vi "HMI_main.vi"() -> ()   [LabVIEW 2018]
uses:
  <vilib>/RAFA Solutions/Harmony UI Controls Kit/String & Path/String Indicator.ctl
  <vilib>/RAFA Solutions/Harmony UI Controls Kit/Boolean/Slide Switch Round.ctl
  Controls/Cluster_HMI_VIFP - 2.ctl
  <vilib>/RAFA Solutions/Harmony UI Controls Kit/Numeric/Horizontal Progress Bar.ctl
  <vilib>/RAFA Solutions/Harmony UI Controls Kit/Numeric/Numeric Indicator.ctl
  <vilib>/RAFA Solutions/Harmony UI Controls Kit/Boolean/Blank Button - Blue.ctl
  <vilib>/RAFA Solutions/Harmony UI Controls Kit/Boolean/Blank Button - Red.ctl
  <vilib>/RAFA Solutions/Harmony UI Controls Kit/Boolean/Blank Button - Grey.ctl
  Controls/Hora y Fecha control.ctl
  Global/MSG.vi
  Global/datos usuario.vi
  <vilib>/addons/database/Connection.llb/DB Tools Open Connec (Path).vi
  Global/estadoGeneradores.vi
  Global/Alarmas_indicadores-LED.vi
  Global/globalEventos.vi
  Global/Demo.vi
  Global/globalGenerador1_HMI.vi
  Global/globalGenerador2_HMI.vi
  Global/globalGenerador3_HMI.vi
  Global/globalGenerador4_HMI.vi
  Global/globalGenerador5_HMI.vi
  Global/globalGenerador6_HMI.vi
  <vilib>/addons/database/NI_Database_API.lvlib
  <vilib>/RAFA Solutions/Harmony UI Controls Kit/Flat UI Design.lvlib
panel:
  out "build":string
  out "fecha y hora":T1
  in  "type specifier VI Refnum (for type only) 3":refnum<vi>
  in  "web_equipo":T2
  in  "type specifier VI Refnum (for type only) 2":refnum<vi>
  out "G6_TRANS":bool caption="Transiente"
  out "G6_SWELL":bool caption="Swell"
  out "G6_SAG":bool caption="Sag"
  out "G5_TRANS":bool caption="Transiente"
  out "G5_SWELL":bool caption="Swell"
  out "G5_SAG":bool caption="Sag"
  out "G4_TRANS":bool caption="Transiente"
  out "G4_SWELL":bool caption="Swell"
  out "G4_SAG":bool caption="Sag"
  out "G3_TRANS":bool caption="Transiente"
  out "G3_SWELL":bool caption="Swell"
  out "G3_SAG":bool caption="Sag"
  out "G2_TRANS":bool caption="Transiente"
  out "G2_SWELL":bool caption="Swell"
  out "G2_SAG":bool caption="Sag"
  out "G1_TRANS":bool caption="Transiente"
  out "G1_SWELL":bool caption="Swell"
  out "G1_SAG":bool caption="Sag"
  in  "type specifier VI Refnum (for type only)":refnum<vi>
  in  "type specifier VI Refnum (for type only)":refnum<vi>
  in  "type specifier VI Refnum (for type only)":refnum<vi>
  in  "configuraciones":T2
  in  "historicos":T2
  in  "eventos":T2
  in  "alarmas":T2
  in  "salir":T3
  in  "type specifier VI Refnum (for type only)":refnum<vi>
  in  "Boolean 6":T4 caption="EMCE_W02"
  out "Estado 6":T5
  in  "Boolean 5":T4 caption="EMCE_W01"
  out "Estado 5":T5
  in  "Boolean 4":T4 caption="EMCE_G04"
  out "Estado 4":T5
  in  "Boolean 3":T4 caption="EMCE_G03"
  out "Estado 3":T5
  in  "Boolean 2":T4 caption="EMCE_G02"
  out "Estado 2":T5
  in  "Boolean 1":T4 caption="EMCE_G01"
  out "Estado 1":T5
  in  "EMCE W02":T6
  in  "EMCE W01":T6
  in  "EMCE G04":T6
  in  "EMCE G03":T6
  in  "EMCE G02":T6
  in  "EMCE G01":T6
  out "Generador6":T7 {"I1" scale=0.0..1200.0; "L1" scale=0.0..600.0; "Factor de Potencia" format="%#.1f"; "Potencia Total [kW]" format="%#.1f"; "Frecuencia [Hz]" format="%#.1f"; "I3" scale=0.0..1200.0; "I2" scale=0.0..1200.0; "L3" scale=0.0..600.0; "L2" scale=0.0..600.0}
  out "Generador5":T7 {"I1" scale=0.0..1200.0; "L1" scale=0.0..600.0; "Factor de Potencia" format="%#.1f"; "Potencia Total [kW]" format="%#.1f"; "Frecuencia [Hz]" format="%#.1f"; "I3" scale=0.0..1200.0; "I2" scale=0.0..1200.0; "L3" scale=0.0..600.0; "L2" scale=0.0..600.0}
  out "Generador4":T7 {"I1" scale=0.0..1200.0; "L1" scale=0.0..600.0; "Factor de Potencia" format="%#.1f"; "Potencia Total [kW]" format="%#.1f"; "Frecuencia [Hz]" format="%#.1f"; "I3" scale=0.0..1200.0; "I2" scale=0.0..1200.0; "L3" scale=0.0..600.0; "L2" scale=0.0..600.0}
  out "Generador3":T7 {"I1" scale=0.0..1200.0; "L1" scale=0.0..600.0; "Factor de Potencia" format="%#.1f"; "Potencia Total [kW]" format="%#.1f"; "Frecuencia [Hz]" format="%#.1f"; "I3" scale=0.0..1200.0; "I2" scale=0.0..1200.0; "L3" scale=0.0..600.0; "L2" scale=0.0..600.0}
  out "Generador2":T7 {"I1" scale=0.0..1200.0; "L1" scale=0.0..600.0; "Factor de Potencia" format="%#.1f"; "Potencia Total [kW]" format="%#.1f"; "Frecuencia [Hz]" format="%#.1f"; "I3" scale=0.0..1200.0; "I2" scale=0.0..1200.0; "L3" scale=0.0..600.0; "L2" scale=0.0..600.0}
  out "Generador1":T7 {"I1" scale=0.0..1200.0; "L1" scale=0.0..600.0; "Factor de Potencia" format="%#.1f"; "Potencia Total [kW]" format="%#.1f"; "Frecuencia [Hz]" format="%#.1f"; "I3" scale=0.0..1200.0; "I2" scale=0.0..1200.0; "L3" scale=0.0..600.0; "L2" scale=0.0..600.0}
  out "Eventos":T5
  # "SMCE"
  # "Sistema de Monitoreo de Calidad de Energía"
  # "POPA"
  # "PROA"
  # "K2"
  # "K1"
  # "RK2"
  # "RK1"
  # "VOLTAJES [Vrms]"
  # "CORRIENTES [Arms]"
  # "VOLTAJES [Vrms]"
  # "CORRIENTES [Arms]"
  # "VOLTAJES [Vrms]"
  # "CORRIENTES [Arms]"
  # "VOLTAJES [Vrms]"
  # "CORRIENTES [Arms]"
  # "VOLTAJES [Vrms]"
  # "CORRIENTES [Arms]"
  # "VOLTAJES [Vrms]"
  # "CORRIENTES [Arms]"
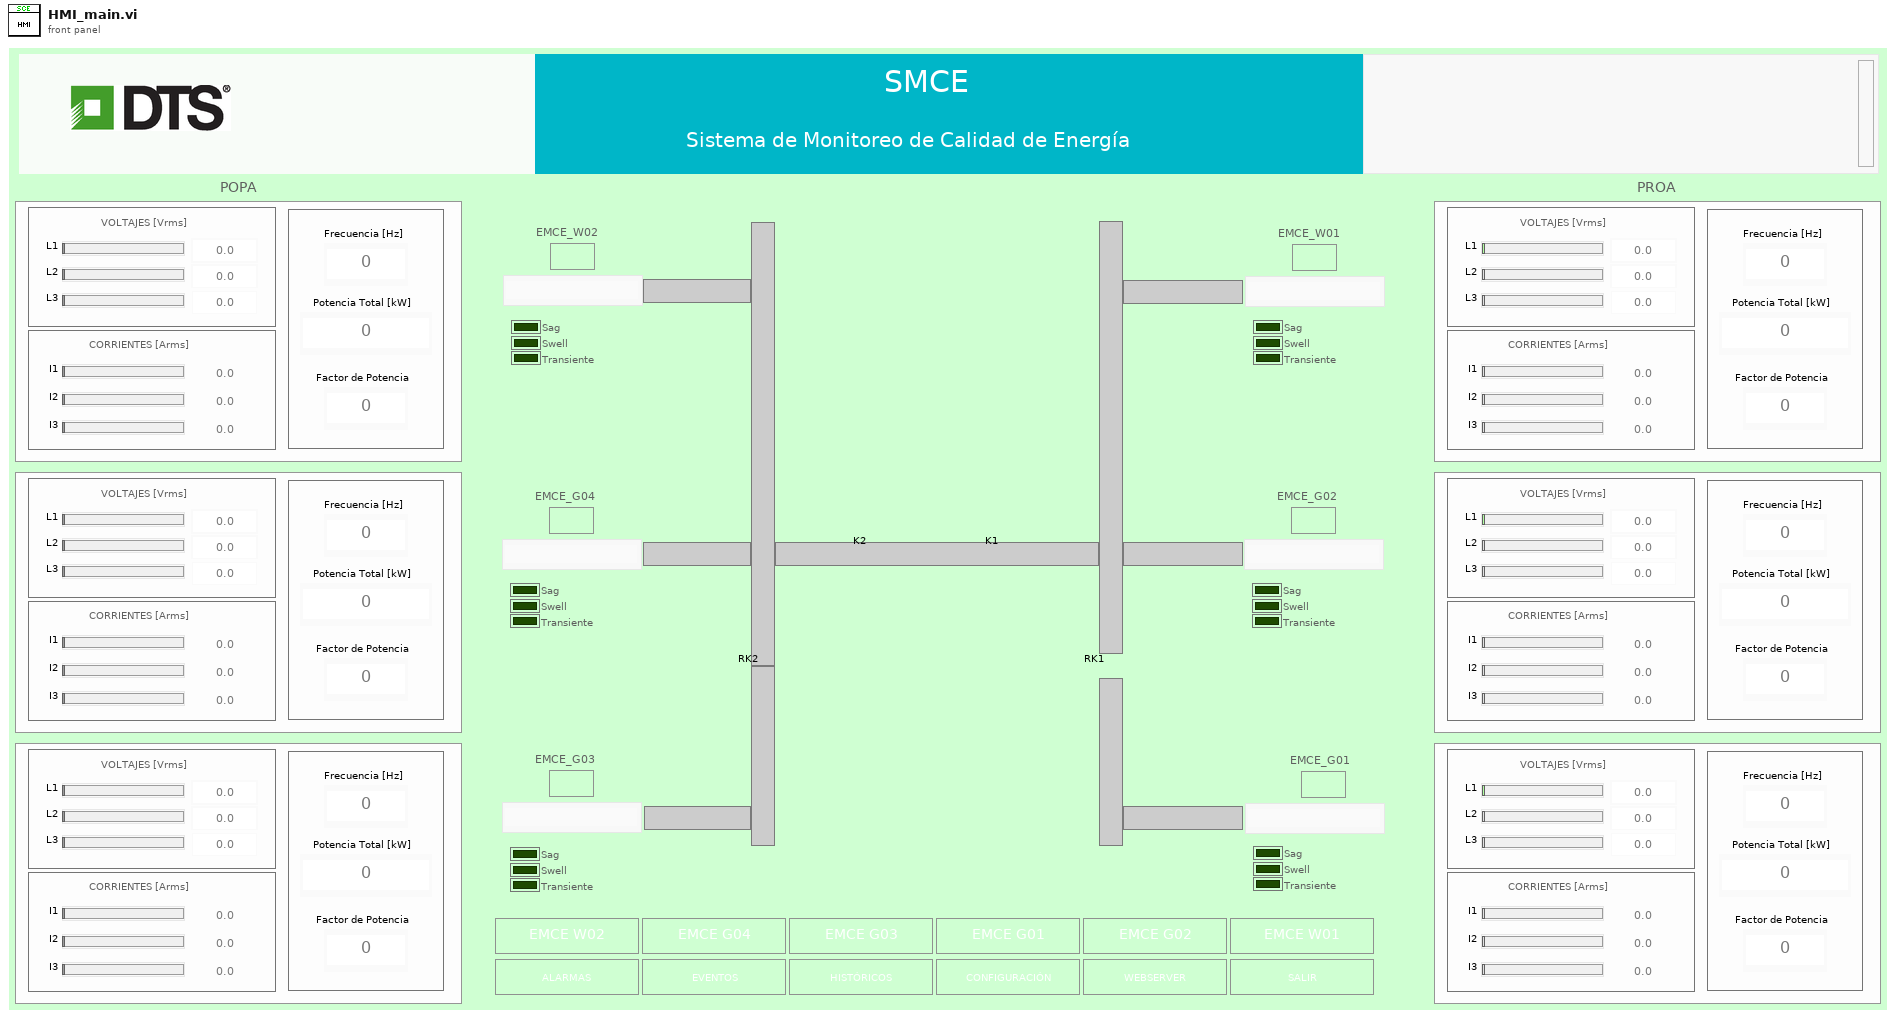
[diagram p1: front panel]
types:
  T1 = typedef "Hora y Fecha control.ctl" = cluster{"fecha":string, "dia semana":string, "fecha 2":string}
  T2 = typedef "Flat UI Design.lvlib/Blank Button - Grey.ctl" = bool
  T3 = typedef "Flat UI Design.lvlib/Blank Button - Red.ctl" = bool
  T4 = typedef "Flat UI Design.lvlib/Slide Switch Round.ctl" = bool
  T5 = typedef "Flat UI Design.lvlib/String Indicator.ctl" = string
  T6 = typedef "Flat UI Design.lvlib/Blank Button - Blue.ctl" = bool
  T7 = typedef "Cluster_HMI_VIFP - 2.ctl" = cluster{"L2":T8, "L3":T8, "I2":T8, "I3":T8, "Frecuencia [Hz]":T9, "Potencia Total [kW]":T9, "Factor de Potencia":T9, "L1":T8, "I1":T8}
  T8 = typedef "Flat UI Design.lvlib/Horizontal Progress Bar.ctl" = sgl
  T9 = typedef "Flat UI Design.lvlib/Numeric Indicator.ctl" = sgl
  T10 = enum8{"Enabled", "Disabled", "Disabled and Grayed Out"}
  T11 = typedef "NI_Database_API.lvlib/Conn ObjectReference.ctl" = refnum<k1>
  T12 = typedef "Equipos_Medicion_cluster.ctl" = cluster{"ID_EQUIPO":i32, "IP_EQUIPO":string, "NOMBRE_EQUIPO":string, "ESTADO_EQUIPO":string, "DESCRIPCION":string, "ID_MEDICION":i32, "ESTADO_MEDICION":string, "TIEMPO_MEDICION":string}
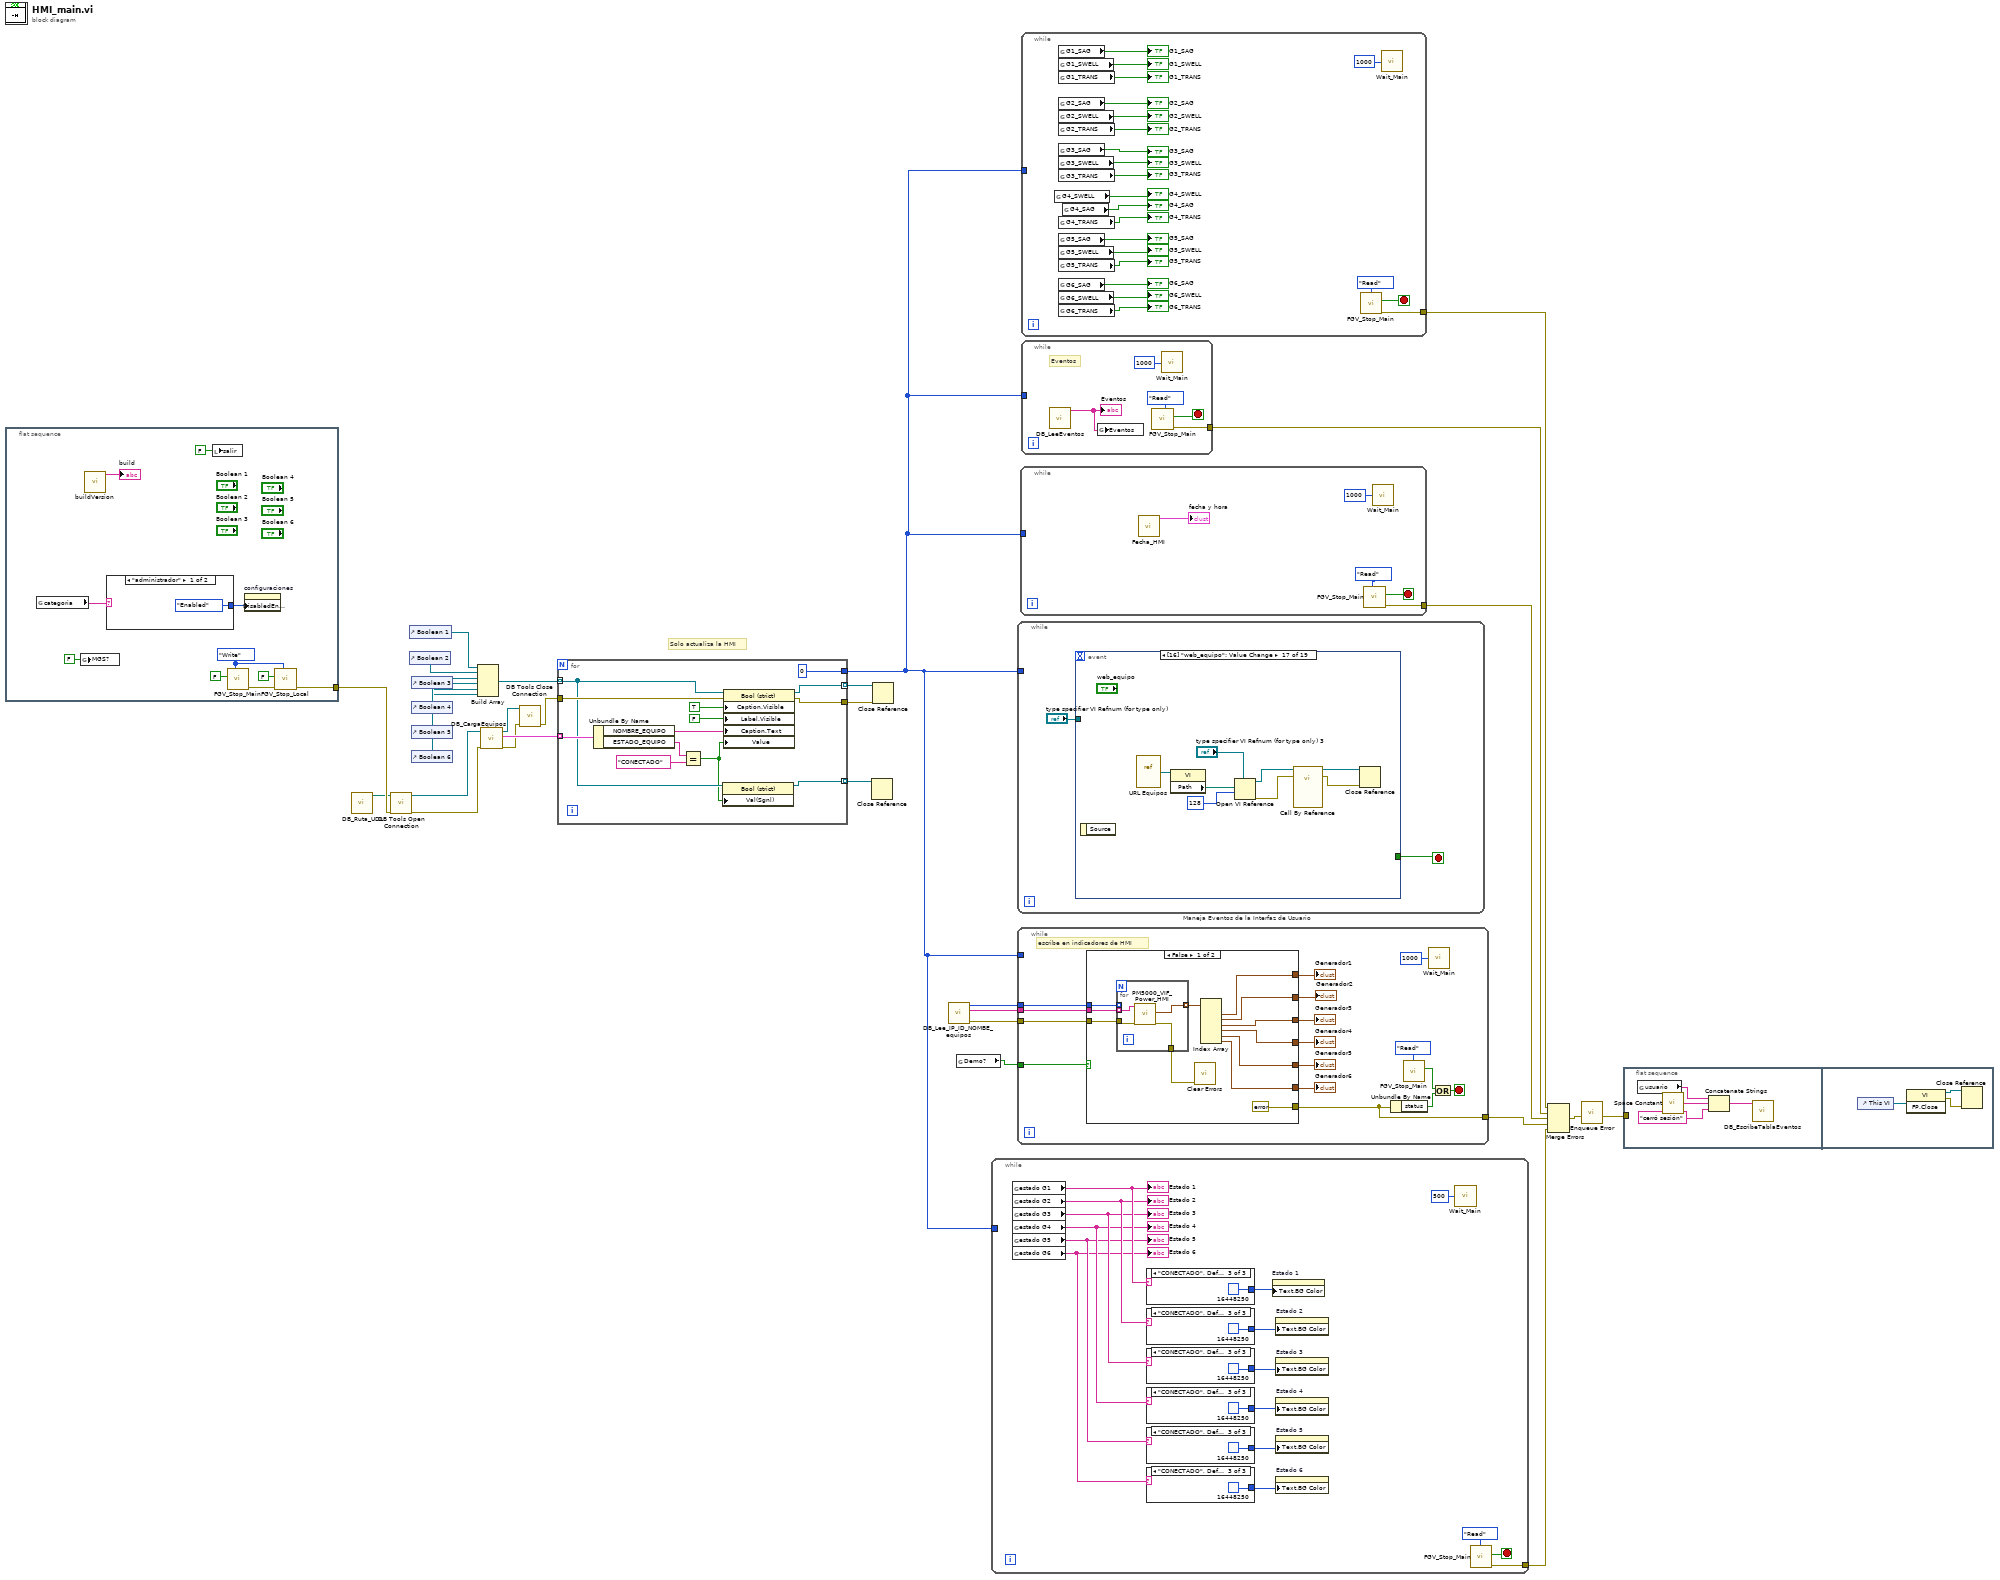
[diagram p0: block diagram]
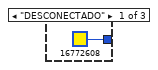
[diagram p2: hidden frame]
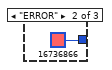
[diagram p3: hidden frame]
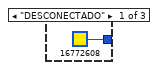
[diagram p4: hidden frame]
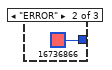
[diagram p5: hidden frame]
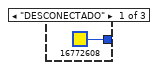
[diagram p6: hidden frame]
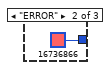
[diagram p7: hidden frame]
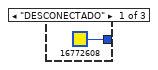
[diagram p8: hidden frame]
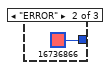
[diagram p9: hidden frame]
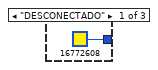
[diagram p10: hidden frame]
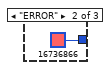
[diagram p11: hidden frame]
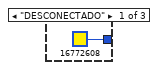
[diagram p12: hidden frame]
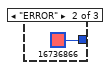
[diagram p13: hidden frame]
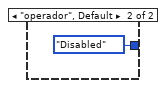
[diagram p14: hidden frame]
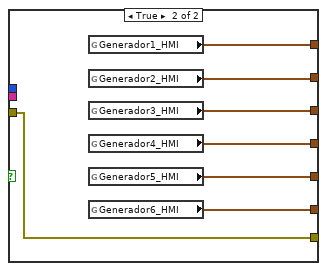
[diagram p15: hidden frame]
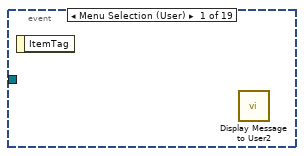
[diagram p16: hidden frame]
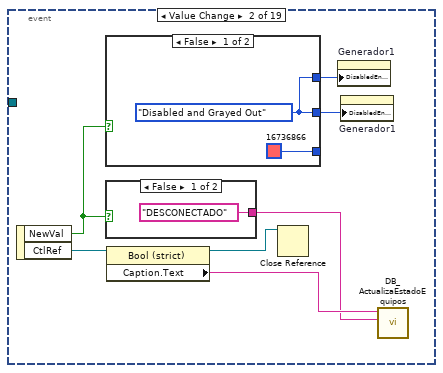
[diagram p17: hidden frame]
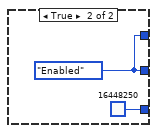
[diagram p18: hidden frame]
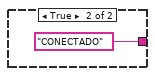
[diagram p19: hidden frame]
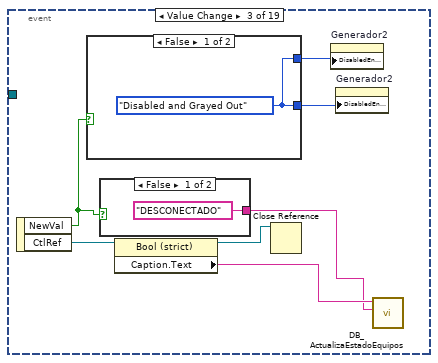
[diagram p20: hidden frame]
diagram:
  # "Solo actualiza la HMI"
  n1 = flat-sequence {
    tunnel: [w35] -> w19
    frame #0 {
      w38 = enum16{"Read", "Write"}."Write" ("Action")
      n2 = global read "datos usuario.vi" "categoria"() -> (w33:string)
      n3 = global write "MSG.vi" "MGS?"(FALSE ("MGS?")) -> ()
      n4 = call "buildVersion.vi"() -> ("build"=→"build":string)  [unwired: 11 in]
      n5 = case shown="\"administrador\"" w33 {
        tunnel: [T10."Enabled" ("Disabled") T10."Disabled" ("Disabled")] -> w34
        frame "administrador" {
        }
        frame "operador", Default {
        }
      }
      n6 = local write "salir"(T3 FALSE ("salir")) -> ()
      n7 = call "FGV_Stop_Main.vi"("Action"=w38, "Var In"=FALSE) -> ("Error Out"=w39:errorcluster)  [unwired: 8 in, 1 out]
      n8 = property on="configuraciones" class="Bool"("DisabledEnum"=w34) -> ()  [unwired: 2 in, 2 out]
      n9 = call "FGV_Stop_Local.vi"("Action"=w38, "Error In (no error)"=w39, "Var In"=FALSE) -> ("Error Out"=w35:errorcluster)  [unwired: 7 in, 1 out]
    }
  }
  n10 = call "DB_Ruta_UDL.vi"() -> ("UDL ruta"=w18:path)  [unwired: 11 in]
  n11 = call-poly <vilib>:"DB Tools Open Connection.vi"("error in (no error)"=w19, "connection information"=w18) -> ("error out"=w21:errorcluster, "connection reference"=w22:T11)  [unwired: 6 in]
  n12 = control-ref of="Boolean 2"() -> (w30:refnum<vi>)
  n13 = control-ref of="Boolean 1"() -> (w24:refnum<vi>)
  n14 = control-ref of="Boolean 3"() -> (w29:refnum<vi>)
  n15 = control-ref of="Boolean 4"() -> (w28:refnum<vi>)
  n16 = control-ref of="Boolean 5"() -> (w27:refnum<vi>)
  n17 = control-ref of="Boolean 6"() -> (w26:refnum<vi>)
  n18 = Build Array(w24, w30, w29, w28, w27, w26) -> (w25:refnum<vi>[])
  n19 = call "DB_CargaEquipos.vi"("error in (no error)"=w21, "db in"=w22) -> ("error out"=w12:errorcluster, "Equipos_out"=w23:T12[], "db out"=w20:T11)  [unwired: 2 in, 5 out]
  n20 = call <vilib>:"DB Tools Close Connection.vi"("error in (no error)"=w12, "connection reference"=w20) -> ("error out"=w11:errorcluster)  [unwired: 5 in]
  n21 = for {
    tunnel: w23 -> [w52] mode=indexing
    tunnel: w25 -> [w45] mode=indexing
    tunnel: [0] -> w2
    tunnel: [w50] -> w17
    tunnel: [w49] -> w16 mode=indexing
    tunnel: w11 -> [w48]
    tunnel: [w43] -> w4 mode=indexing
    n22 = Unbundle By Name(w52) -> ("NOMBRE_EQUIPO"=w47:string, "ESTADO_EQUIPO"=w46:string)
    n23 = Equal?(x=w46, y="CONECTADO") -> (x = y?=w44:bool)
    n24 = property class="Bool (strict)"(reference=w45, "Val(Sgnl)"=w44) -> (reference out=w43:refnum<vi>)  [unwired: 1 in, 1 out]
    n25 = property class="Bool (strict)"(reference=w45, error in=w48, "Caption.Visible"=TRUE ("Label.Visible"), "Label.Visible"=FALSE ("Caption.Visible"), "Caption.Text"=w47, "Value"=w44) -> (reference out=w49:refnum<vi>, error out=w50:errorcluster)
  }
  n26 = Close Reference(reference=w4) -> ()  [unwired: 1 in, 1 out]
  n27 = Close Reference(reference=w16, error in (no error)=w17) -> ()  [unwired: 1 out]
  n28 = call "DB_Lee_IP_ID_NOMBE_equipos.vi"() -> ("error out"=w15:errorcluster, "IP_EQUIPO"=w14:string[], "ID_EQUIPO"=w13:i32[])  [unwired: 8 in, 1 out]
  n29 = global read "Demo.vi" "Demo?"() -> (w1:bool)
  n30 = while {
    tunnel: [w56] -> w3
    tunnel: w2 -> [_]
    stop <- w70 stop-if-true
    n31 = global read "estadoGeneradores.vi" "estado G1"() -> (w68:string)
    "Estado 1" <- w68
    n32 = global read "estadoGeneradores.vi" "estado G2"() -> (w66:string)
    "Estado 2" <- w66
    n33 = global read "estadoGeneradores.vi" "estado G3"() -> (w65:string)
    "Estado 3" <- w65
    n34 = global read "estadoGeneradores.vi" "estado G4"() -> (w64:string)
    "Estado 4" <- w64
    n35 = global read "estadoGeneradores.vi" "estado G5"() -> (w63:string)
    "Estado 5" <- w63
    n36 = global read "estadoGeneradores.vi" "estado G6"() -> (w62:string)
    "Estado 6" <- w62
    n37 = case shown="\"CONECTADO\", Default" w68 {
      tunnel: [u32 16772608 u32 16736866 u32 16448250] -> w67
      frame "DESCONECTADO" {
      }
      frame "ERROR" {
      }
      frame "CONECTADO", Default {
      }
    }
    n38 = case shown="\"CONECTADO\", Default" w66 {
      tunnel: [u32 16772608 u32 16736866 u32 16448250] -> w61
      frame "DESCONECTADO" {
      }
      frame "ERROR" {
      }
      frame "CONECTADO", Default {
      }
    }
    n39 = case shown="\"CONECTADO\", Default" w65 {
      tunnel: [u32 16772608 u32 16736866 u32 16448250] -> w60
      frame "DESCONECTADO" {
      }
      frame "ERROR" {
      }
      frame "CONECTADO", Default {
      }
    }
    n40 = case shown="\"CONECTADO\", Default" w64 {
      tunnel: [u32 16772608 u32 16736866 u32 16448250] -> w59
      frame "DESCONECTADO" {
      }
      frame "ERROR" {
      }
      frame "CONECTADO", Default {
      }
    }
    n41 = case shown="\"CONECTADO\", Default" w63 {
      tunnel: [u32 16772608 u32 16736866 u32 16448250] -> w58
      frame "DESCONECTADO" {
      }
      frame "ERROR" {
      }
      frame "CONECTADO", Default {
      }
    }
    n42 = case shown="\"CONECTADO\", Default" w62 {
      tunnel: [u32 16772608 u32 16736866 u32 16448250] -> w57
      frame "DESCONECTADO" {
      }
      frame "ERROR" {
      }
      frame "CONECTADO", Default {
      }
    }
    n43 = property on="Estado 1" class="Str (strict)"("Text.BG Color"=w67) -> ()  [unwired: 2 in, 2 out]
    n44 = property on="Estado 2" class="Str (strict)"("Text.BG Color"=w61) -> ()  [unwired: 2 in, 2 out]
    n45 = property on="Estado 3" class="Str (strict)"("Text.BG Color"=w60) -> ()  [unwired: 2 in, 2 out]
    n46 = property on="Estado 4" class="Str (strict)"("Text.BG Color"=w59) -> ()  [unwired: 2 in, 2 out]
    n47 = property on="Estado 5" class="Str (strict)"("Text.BG Color"=w58) -> ()  [unwired: 2 in, 2 out]
    n48 = property on="Estado 6" class="Str (strict)"("Text.BG Color"=w57) -> ()  [unwired: 2 in, 2 out]
    n49 = call "Wait_Main.vi"("Wait time (msec)"=u32 500 ("milliseconds to wait")) -> ()  [unwired: 5 in]
    n50 = call "FGV_Stop_Main.vi"("Action"=enum16{"Read", "Write"}."Read") -> ("Error Out"=w56:errorcluster, "Var Out"=w70:bool)  [unwired: 9 in]
  }
  n51 = while "Maneja Eventos de la Interfaz de Usuario" {
    tunnel: w2 -> [_]
    stop <- w91 stop-if-true
    n52 = event shown="[16] \"web_equipo\": Value Change" {
      selector: _ -> [_ _ _ _ _ _ _ _ _ _ _ _ _ _ _ _ _ _ _]
      dyn-events: _ -> [_ _ _ _ _ _ _ _ _ _ _ _ _ _ _ _ _ _ _]
      timeout: _ -> [_ _ _ _ _ _ _ _ _ _ _ _ _ _ _ _ _ _ _]
      tunnel: [_ _ _ _ _ _ _ w167 _ _ _ _ _ _ _ _ _ _ _] -> w91
      tunnel: "type specifier VI Refnum (for type only)" -> [_ _ _ _ _ _ _ _ w178 w191 w203 w215 w227 w239 _ _ _ _ _]
      event Menu Selection (User) {
        n53 = event-data() -> ()  [unwired: 2 out]
        n54 = call "Display Message to User2"() -> ()  [unwired: 10 in, 2 out]
      }
      event Value Change {
        n55 = event-data() -> ("NewVal"=w96:T4, "CtlRef"=w98:refnum<vi>)  [unwired: 1 out]
        n56 = case shown="False" w96 {
          tunnel: [w99 w101] -> w97
          tunnel: [u32 16736866 u32 16448250] -> _
          tunnel: [w99 w101] -> w95
          frame False {
            w99 = T10."Disabled and Grayed Out" ("Disabled")
          }
          frame True {
            w101 = T10."Enabled" ("Disabled")
          }
        }
        n57 = case shown="False" w96 {
          tunnel: ["DESCONECTADO" ("y") "CONECTADO" ("y")] -> w92
          frame False {
          }
          frame True {
          }
        }
        n58 = property class="Bool (strict)"(reference=w98) -> (reference out=w94:refnum<vi>, "Caption.Text"=w93:string)  [unwired: 1 in, 1 out]
        n59 = Close Reference(reference=w94) -> ()  [unwired: 1 in, 1 out]
        n60 = property on="Generador1" class="Bool"("DisabledEnum"=w95) -> ()  [unwired: 2 in, 2 out]
        n61 = property on="Generador1" class="Clust (strict)"("DisabledEnum"=w97) -> ()  [unwired: 2 in, 2 out]
        n62 = call "DB_ActualizaEstadoEquipos.vi"("ESTADO_EQUIPO"=w92, "NOMBRE_EQUIPO"=w93) -> ()  [unwired: 9 in, 1 out]
      }
      event Value Change {
        n63 = event-data() -> ("NewVal"=w110:T4, "CtlRef"=w111:refnum<vi>)  [unwired: 1 out]
        n64 = case shown="False" w110 {
          tunnel: [w112 w113] -> w109
          tunnel: [w112 w113] -> w108
          frame False {
            w112 = T10."Disabled and Grayed Out" ("Disabled")
          }
          frame True {
            (unwired) u32 16448250
            w113 = T10."Enabled" ("Disabled")
          }
        }
        n65 = case shown="False" w110 {
          tunnel: ["DESCONECTADO" ("y") "CONECTADO" ("y")] -> w105
          frame False {
          }
          frame True {
          }
        }
        n66 = property class="Bool (strict)"(reference=w111) -> (reference out=w107:refnum<vi>, "Caption.Text"=w106:string)  [unwired: 1 in, 1 out]
        n67 = Close Reference(reference=w107) -> ()  [unwired: 1 in, 1 out]
        n68 = property on="Generador2" class="Clust (strict)"("DisabledEnum"=w108) -> ()  [unwired: 2 in, 2 out]
        n69 = property on="Generador2" class="Bool"("DisabledEnum"=w109) -> ()  [unwired: 2 in, 2 out]
        n70 = call "DB_ActualizaEstadoEquipos.vi"("ESTADO_EQUIPO"=w105, "NOMBRE_EQUIPO"=w106) -> ()  [unwired: 9 in, 1 out]
      }
      event Value Change {
        n71 = event-data() -> ("NewVal"=w120:T4, "CtlRef"=w122:refnum<vi>)  [unwired: 1 out]
        n72 = case shown="False" w120 {
          tunnel: [w124 w125] -> w121
          tunnel: [u32 16736866 u32 16448250] -> _
          tunnel: [w124 w125] -> w116
          frame False {
            w124 = T10."Disabled and Grayed Out" ("Disabled")
          }
          frame True {
            w125 = T10."Enabled" ("Disabled")
          }
        }
        n73 = case shown="True" w120 {
          tunnel: ["DESCONECTADO" ("y") "CONECTADO" ("y")] -> w117
          frame False {
          }
          frame True {
          }
        }
        n74 = property class="Bool (strict)"(reference=w122) -> (reference out=w119:refnum<vi>, "Caption.Text"=w118:string)  [unwired: 1 in, 1 out]
        n75 = Close Reference(reference=w119) -> ()  [unwired: 1 in, 1 out]
        n76 = property on="Generador3" class="Bool"("DisabledEnum"=w121) -> ()  [unwired: 2 in, 2 out]
        n77 = property on="Generador3" class="Clust (strict)"("DisabledEnum"=w116) -> ()  [unwired: 2 in, 2 out]
        n78 = call "DB_ActualizaEstadoEquipos.vi"("ESTADO_EQUIPO"=w117, "NOMBRE_EQUIPO"=w118) -> ()  [unwired: 9 in, 1 out]
      }
      event Value Change {
        n79 = event-data() -> ("NewVal"=w134:T4, "CtlRef"=w135:refnum<vi>)  [unwired: 1 out]
        n80 = case shown="False" w134 {
          tunnel: [w137 w138] -> w132
          tunnel: [u32 16736866 u32 16448250] -> _
          tunnel: [w137 w138] -> w133
          frame False {
            w137 = T10."Disabled and Grayed Out" ("Disabled")
          }
          frame True {
            w138 = T10."Enabled" ("Disabled")
          }
        }
        n81 = case shown="False" w134 {
          tunnel: ["DESCONECTADO" ("y") "CONECTADO" ("y")] -> w129
          frame False {
          }
          frame True {
          }
        }
        n82 = property class="Bool (strict)"(reference=w135) -> (reference out=w131:refnum<vi>, "Caption.Text"=w130:string)  [unwired: 1 in, 1 out]
        n83 = Close Reference(reference=w131) -> ()  [unwired: 1 in, 1 out]
        n84 = property on="Generador4" class="Clust (strict)"("DisabledEnum"=w133) -> ()  [unwired: 2 in, 2 out]
        n85 = property on="Generador4" class="Bool"("DisabledEnum"=w132) -> ()  [unwired: 2 in, 2 out]
        n86 = call "DB_ActualizaEstadoEquipos.vi"("ESTADO_EQUIPO"=w129, "NOMBRE_EQUIPO"=w130) -> ()  [unwired: 9 in, 1 out]
      }
      event Value Change {
        n87 = event-data() -> ("NewVal"=w147:T4, "CtlRef"=w148:refnum<vi>)  [unwired: 1 out]
        n88 = case shown="True" w147 {
          tunnel: [w149 w150] -> w145
          tunnel: [w149 w150] -> w146
          frame False {
            w149 = T10."Disabled and Grayed Out" ("Disabled")
          }
          frame True {
            (unwired) u32 16448250
            w150 = T10."Enabled" ("Disabled")
          }
        }
        n89 = case shown="False" w147 {
          tunnel: ["DESCONECTADO" ("y") "CONECTADO" ("y")] -> w142
          frame False {
          }
          frame True {
          }
        }
        n90 = property class="Bool (strict)"(reference=w148) -> (reference out=w144:refnum<vi>, "Caption.Text"=w143:string)  [unwired: 1 in, 1 out]
        n91 = Close Reference(reference=w144) -> ()  [unwired: 1 in, 1 out]
        n92 = property on="Generador5" class="Clust (strict)"("DisabledEnum"=w146) -> ()  [unwired: 2 in, 2 out]
        n93 = property on="Generador5" class="Bool"("DisabledEnum"=w145) -> ()  [unwired: 2 in, 2 out]
        n94 = call "DB_ActualizaEstadoEquipos.vi"("ESTADO_EQUIPO"=w142, "NOMBRE_EQUIPO"=w143) -> ()  [unwired: 9 in, 1 out]
      }
      event Value Change {
        n95 = event-data() -> ("NewVal"=w158:T4, "CtlRef"=w159:refnum<vi>)  [unwired: 1 out]
        n96 = case shown="False" w158 {
          tunnel: ["DESCONECTADO" ("y") "CONECTADO" ("y")] -> w153
          frame False {
          }
          frame True {
          }
        }
        n97 = case shown="False" w158 {
          tunnel: [w161 w162] -> w156
          tunnel: [u32 16736866 u32 16448250] -> _
          tunnel: [w161 w162] -> w157
          frame False {
            w161 = T10."Disabled and Grayed Out" ("Disabled")
          }
          frame True {
            w162 = T10."Enabled" ("Disabled")
          }
        }
        n98 = property class="Bool (strict)"(reference=w159) -> (reference out=w155:refnum<vi>, "Caption.Text"=w154:string)  [unwired: 1 in, 1 out]
        n99 = Close Reference(reference=w155) -> ()  [unwired: 1 in, 1 out]
        n100 = property on="Generador6" class="Clust (strict)"("DisabledEnum"=w157) -> ()  [unwired: 2 in, 2 out]
        n101 = property on="Generador6" class="Bool"("DisabledEnum"=w156) -> ()  [unwired: 2 in, 2 out]
        n102 = call "DB_ActualizaEstadoEquipos.vi"("ESTADO_EQUIPO"=w153, "NOMBRE_EQUIPO"=w154) -> ()  [unwired: 9 in, 1 out]
      }
      event Value Change {
        w170 = enum16{"Read", "Write"}."Write" ("Action")
        # "detiene el MAIN\ny todos los demas\nprocesos"
        n103 = event-data() -> ()  [unwired: 4 out]
        n104 = global read "MSG.vi" "MGS?"() -> (w166:bool)
        n105 = case shown="True" w166 {
          tunnel: [w174 TRUE] -> w167
          frame False {
            n106 = call "Display Message to User"() -> ("SI"=w171:bool)  [unwired: 10 in, 1 out]
            n107 = Select(t=TRUE, s=w171, f=FALSE) -> (s? t:f=w174:bool)
          }
          frame True {
            # "se cierra la aplicacion\nsin perguntar"
          }
        }
        n108 = call "FGV_Stop_Main.vi"("Action"=w170, "Var In"=w167) -> ("Error Out"=w169:errorcluster)  [unwired: 8 in, 1 out]
        n109 = call "FGV_Stop_Local.vi"("Action"=w170, "Error In (no error)"=w169, "Var In"=TRUE) -> ()  [unwired: 7 in, 2 out]
      }
      event Value Change {
        n110 = event-data() -> ()  [unwired: 2 out]
        n111 = vi-ref "Graficas.vi"() -> (w189:refnum<vi>)
        n112 = property class="VI"(reference=w189) -> ("Path"=w184:path)  [unwired: 1 in, 2 out]
        n113 = call "DB_Lee_IP_ID_NOMBE_equipos.vi"() -> ("error out"=w176:errorcluster, "ID_EQUIPO"=w181:i32[])  [unwired: 8 in, 2 out]
        n114 = Index Array(array=w181, index=0) -> (element=w179:i32)
        n115 = Open VI Reference(type specifier VI Refnum (for type only)=w178, vi path=w184, options=128) -> (vi reference=w183:refnum<vi>, error out=w188:errorcluster)  [unwired: 3 in]
        n116 = call-by-ref "?"(reference=w183, error in=w188, "ID_EQUIPO"=w179, "Generador in"="EMCE G01" ("Var In")) -> (reference out=w187:refnum<vi>, error out=w186:errorcluster)  [unwired: 1 in]
        n117 = Close Reference(reference=w187, error in (no error)=w186) -> (error out=w185:errorcluster)
        n118 = Merge Errors(w185, w176) -> ()  [unwired: 1 out]
      }
      event Value Change {
        n119 = event-data() -> ()  [unwired: 2 out]
        n120 = vi-ref "Graficas.vi"() -> (w201:refnum<vi>)
        n121 = property class="VI"(reference=w201) -> ("Path"=w197:path)  [unwired: 1 in, 2 out]
        n122 = call "DB_Lee_IP_ID_NOMBE_equipos.vi"() -> ("ID_EQUIPO"=w194:i32[])  [unwired: 8 in, 3 out]
        n123 = Index Array(array=w194, index=1) -> (element=w192:i32)
        n124 = Open VI Reference(type specifier VI Refnum (for type only)=w191, vi path=w197, options=128) -> (vi reference=w196:refnum<vi>, error out=w200:errorcluster)  [unwired: 3 in]
        n125 = call-by-ref "?"(reference=w196, error in=w200, "ID_EQUIPO"=w192, "Generador in"="EMCE G02" ("Var In")) -> (reference out=w199:refnum<vi>, error out=w198:errorcluster)  [unwired: 1 in]
        n126 = Close Reference(reference=w199, error in (no error)=w198) -> ()  [unwired: 1 out]
      }
      event Value Change {
        n127 = event-data() -> ()  [unwired: 2 out]
        n128 = vi-ref "Graficas.vi"() -> (w213:refnum<vi>)
        n129 = property class="VI"(reference=w213) -> ("Path"=w209:path)  [unwired: 1 in, 2 out]
        n130 = call "DB_Lee_IP_ID_NOMBE_equipos.vi"() -> ("ID_EQUIPO"=w206:i32[])  [unwired: 8 in, 3 out]
        n131 = Index Array(array=w206, index=2) -> (element=w204:i32)
        n132 = Open VI Reference(type specifier VI Refnum (for type only)=w203, vi path=w209, options=128) -> (vi reference=w208:refnum<vi>, error out=w212:errorcluster)  [unwired: 3 in]
        n133 = call-by-ref "?"(reference=w208, error in=w212, "ID_EQUIPO"=w204, "Generador in"="EMCE G03" ("Var In")) -> (reference out=w211:refnum<vi>, error out=w210:errorcluster)  [unwired: 1 in]
        n134 = Close Reference(reference=w211, error in (no error)=w210) -> ()  [unwired: 1 out]
      }
      event Value Change {
        n135 = event-data() -> ()  [unwired: 2 out]
        n136 = vi-ref "Graficas.vi"() -> (w225:refnum<vi>)
        n137 = property class="VI"(reference=w225) -> ("Path"=w221:path)  [unwired: 1 in, 2 out]
        n138 = call "DB_Lee_IP_ID_NOMBE_equipos.vi"() -> ("ID_EQUIPO"=w218:i32[])  [unwired: 8 in, 3 out]
        n139 = Index Array(array=w218, index=3) -> (element=w216:i32)
        n140 = Open VI Reference(type specifier VI Refnum (for type only)=w215, vi path=w221, options=128) -> (vi reference=w220:refnum<vi>, error out=w224:errorcluster)  [unwired: 3 in]
        n141 = call-by-ref "?"(reference=w220, error in=w224, "ID_EQUIPO"=w216, "Generador in"="EMCE G04" ("Var In")) -> (reference out=w223:refnum<vi>, error out=w222:errorcluster)  [unwired: 1 in]
        n142 = Close Reference(reference=w223, error in (no error)=w222) -> ()  [unwired: 1 out]
      }
      event Value Change {
        n143 = event-data() -> ()  [unwired: 2 out]
        n144 = vi-ref "Graficas.vi"() -> (w237:refnum<vi>)
        n145 = property class="VI"(reference=w237) -> ("Path"=w233:path)  [unwired: 1 in, 2 out]
        n146 = call "DB_Lee_IP_ID_NOMBE_equipos.vi"() -> ("ID_EQUIPO"=w230:i32[])  [unwired: 8 in, 3 out]
        n147 = Index Array(array=w230, index=4) -> (element=w228:i32)
        n148 = Open VI Reference(type specifier VI Refnum (for type only)=w227, vi path=w233, options=128) -> (vi reference=w232:refnum<vi>, error out=w236:errorcluster)  [unwired: 3 in]
        n149 = call-by-ref "?"(reference=w232, error in=w236, "ID_EQUIPO"=w228, "Generador in"="EMCE W01" ("Var In")) -> (reference out=w235:refnum<vi>, error out=w234:errorcluster)  [unwired: 1 in]
        n150 = Close Reference(reference=w235, error in (no error)=w234) -> ()  [unwired: 1 out]
      }
      event Value Change {
        n151 = event-data() -> ()  [unwired: 2 out]
        n152 = vi-ref "Graficas.vi"() -> (w249:refnum<vi>)
        n153 = property class="VI"(reference=w249) -> ("Path"=w245:path)  [unwired: 1 in, 2 out]
        n154 = call "DB_Lee_IP_ID_NOMBE_equipos.vi"() -> ("ID_EQUIPO"=w242:i32[])  [unwired: 8 in, 3 out]
        n155 = Index Array(array=w242, index=5) -> (element=w240:i32)
        n156 = Open VI Reference(type specifier VI Refnum (for type only)=w239, vi path=w245, options=128) -> (vi reference=w244:refnum<vi>, error out=w248:errorcluster)  [unwired: 3 in]
        n157 = call-by-ref "?"(reference=w244, error in=w248, "ID_EQUIPO"=w240, "Generador in"="EMCE W02" ("Var In")) -> (reference out=w247:refnum<vi>, error out=w246:errorcluster)  [unwired: 1 in]
        n158 = Close Reference(reference=w247, error in (no error)=w246) -> ()  [unwired: 1 out]
      }
      event Value Change {
        n159 = event-data() -> ()  [unwired: 4 out]
        n160 = vi-ref "Historicos.vi"() -> (w257:refnum<vi>)
        n161 = property class="VI"(reference=w257) -> ("Path"=w253:path)  [unwired: 1 in, 2 out]
        n162 = Open VI Reference(type specifier VI Refnum (for type only)="type specifier VI Refnum (for type only)", vi path=w253, options=128) -> (vi reference=w252:refnum<vi>, error out=w256:errorcluster)  [unwired: 3 in]
        n163 = call-by-ref "?"(reference=w252, error in=w256) -> (reference out=w255:refnum<vi>, error out=w254:errorcluster)  [unwired: 3 in]
        n164 = Close Reference(reference=w255, error in (no error)=w254) -> ()  [unwired: 1 out]
      }
      event Value Change {
        n165 = event-data() -> ()  [unwired: 4 out]
        n166 = vi-ref "Configuracion.vi"() -> (w265:refnum<vi>)
        n167 = property class="VI"(reference=w265) -> ("Path"=w261:path)  [unwired: 1 in, 2 out]
        n168 = Open VI Reference(type specifier VI Refnum (for type only)="type specifier VI Refnum (for type only) 2", vi path=w261, options=128) -> (vi reference=w259:refnum<vi>, error out=w264:errorcluster)  [unwired: 3 in]
        n169 = call-by-ref "?"(reference=w259, error in=w264) -> (reference out=w263:refnum<vi>, error out=w262:errorcluster)  [unwired: 12 in]
        n170 = Close Reference(reference=w263, error in (no error)=w262) -> ()  [unwired: 1 out]
      }
      event Value Change {
        n171 = event-data() -> ()  [unwired: 2 out]
        n172 = vi-ref "URL Equipos.vi"() -> (w273:refnum<vi>)
        n173 = property class="VI"(reference=w273) -> ("Path"=w269:path)  [unwired: 1 in, 2 out]
        n174 = Open VI Reference(type specifier VI Refnum (for type only)="type specifier VI Refnum (for type only) 3", vi path=w269, options=128) -> (vi reference=w268:refnum<vi>, error out=w272:errorcluster)  [unwired: 3 in]
        n175 = call-by-ref "?"(reference=w268, error in=w272) -> (reference out=w271:refnum<vi>, error out=w270:errorcluster)  [unwired: 12 in]
        n176 = Close Reference(reference=w271, error in (no error)=w270) -> ()  [unwired: 1 out]
      }
      event Value Change {
        n177 = event-data() -> ()  [unwired: 4 out]
        n178 = vi-ref "Eventos.vi"() -> (w281:refnum<vi>)
        n179 = property class="VI"(reference=w281) -> ("Path"=w277:path)  [unwired: 1 in, 2 out]
        n180 = Open VI Reference(type specifier VI Refnum (for type only)="type specifier VI Refnum (for type only)", vi path=w277, options=128) -> (vi reference=w275:refnum<vi>, error out=w280:errorcluster)  [unwired: 3 in]
        n181 = call-by-ref "?"(reference=w275, error in=w280) -> (reference out=w279:refnum<vi>, error out=w278:errorcluster)  [unwired: 3 in]
        n182 = Close Reference(reference=w279, error in (no error)=w278) -> ()  [unwired: 1 out]
      }
      event Value Change {
        n183 = event-data() -> ()  [unwired: 4 out]
        n184 = vi-ref "AlarmasHMI.vi"() -> (w289:refnum<vi>)
        n185 = property class="VI"(reference=w289) -> ("Path"=w285:path)  [unwired: 1 in, 2 out]
        n186 = Open VI Reference(type specifier VI Refnum (for type only)="type specifier VI Refnum (for type only)", vi path=w285, options=128) -> (vi reference=w283:refnum<vi>, error out=w288:errorcluster)  [unwired: 3 in]
        n187 = call-by-ref "?"(reference=w283, error in=w288) -> (reference out=w287:refnum<vi>, error out=w286:errorcluster)  [unwired: 3 in]
        n188 = Close Reference(reference=w287, error in (no error)=w286) -> ()  [unwired: 1 out]
      }
    }
  }
  n189 = while {
    tunnel: w15 -> [w298]
    tunnel: w14 -> [w297]
    tunnel: w13 -> [w296]
    tunnel: [w291] -> w7
    tunnel: w2 -> [_]
    tunnel: w1 -> [w290]
    stop <- w294 stop-if-true
    # "escribe en indicadores de HMI"
    n190 = case shown="False" w290 {
      tunnel: w296 -> [w317 _]
      tunnel: [w316 w328] -> w305
      tunnel: [w315 w327] -> w295
      tunnel: [w314 w326] -> w304
      tunnel: [w313 w325] -> w303
      tunnel: [w312 w324] -> w302
      tunnel: [w311 w323] -> w301
      tunnel: w298 -> [w310 w322]
      tunnel: w297 -> [w309 _]
      tunnel: [errorcluster {"status"=FALSE, "code"=0, "source"=""} ("error out") w322] -> w291
      frame False {
        n191 = for {
          tunnel: w317 -> [_] mode=indexing
          tunnel: w310 -> [w320]
          tunnel: w309 -> [w321] mode=indexing
          tunnel: [w319] -> w308 mode=indexing
          tunnel: [w318] -> w306
          n192 = call "PM5000_VIF_Power_HMI.vi"("error in"=w320, "Network Path"=w321) -> ("error out"=w318:errorcluster, "Generador1"=w319:T7)  [unwired: 7 in, 1 out]
        }
        n193 = call <vilib>:"Clear Errors.vi"("error in (no error)"=w306) -> ()  [unwired: 5 in, 2 out]
        n194 = Index Array(array=w308) -> (element #1=w316:T7, element #2=w315:T7, element #3=w314:T7, element #4=w313:T7, element #5=w312:T7, element #6=w311:T7)  [unwired: 6 in]
      }
      frame True {
        n195 = global read "globalGenerador1_HMI.vi" "Generador1_HMI"() -> (w328:T7)
        n196 = global read "globalGenerador2_HMI.vi" "Generador2_HMI"() -> (w327:T7)
        n197 = global read "globalGenerador3_HMI.vi" "Generador3_HMI"() -> (w326:T7)
        n198 = global read "globalGenerador4_HMI.vi" "Generador4_HMI"() -> (w325:T7)
        n199 = global read "globalGenerador5_HMI.vi" "Generador5_HMI"() -> (w324:T7)
        n200 = global read "globalGenerador6_HMI.vi" "Generador6_HMI"() -> (w323:T7)
      }
    }
    "Generador1" <- w305
    "Generador3" <- w304
    "Generador6" <- w301
    "Generador4" <- w303
    "Generador5" <- w302
    "Generador2" <- w295
    n201 = Unbundle By Name(w291) -> ("status"=w292:bool)
    n202 = call "FGV_Stop_Main.vi"("Action"=enum16{"Read", "Write"}."Read") -> ("Var Out"=w293:bool)  [unwired: 9 in, 1 out]
    n203 = call "Wait_Main.vi"("Wait time (msec)"=u32 1000 ("milliseconds to wait")) -> ()  [unwired: 5 in]
    n204 = Or(x=w293, y=w292) -> (x .or. y?=w294:bool)
  }
  n205 = while {
    tunnel: w2 -> [_]
    tunnel: [w329] -> w8
    stop <- w332 stop-if-true
    n206 = call "Fecha_HMI.vi"() -> ("fecha y hora"=→"fecha y hora":T1)  [unwired: 11 in]
    n207 = call "FGV_Stop_Main.vi"("Action"=enum16{"Read", "Write"}."Read") -> ("Error Out"=w329:errorcluster, "Var Out"=w332:bool)  [unwired: 9 in]
    n208 = call "Wait_Main.vi"("Wait time (msec)"=u32 1000 ("milliseconds to wait")) -> ()  [unwired: 5 in]
  }
  n209 = while {
    tunnel: w2 -> [_]
    tunnel: [w334] -> w10
    stop <- w353 stop-if-true
    n210 = global read "Alarmas_indicadores-LED.vi" "G4_SWELL"() -> (→"G4_SWELL":bool)
    n211 = global read "Alarmas_indicadores-LED.vi" "G1_SAG"() -> (→"G1_SAG":bool)
    n212 = global read "Alarmas_indicadores-LED.vi" "G1_SWELL"() -> (→"G1_SWELL":bool)
    n213 = global read "Alarmas_indicadores-LED.vi" "G1_TRANS"() -> (→"G1_TRANS":bool)
    n214 = global read "Alarmas_indicadores-LED.vi" "G2_SAG"() -> (→"G2_SAG":bool)
    n215 = global read "Alarmas_indicadores-LED.vi" "G2_SWELL"() -> (→"G2_SWELL":bool)
    n216 = global read "Alarmas_indicadores-LED.vi" "G2_TRANS"() -> (→"G2_TRANS":bool)
    n217 = global read "Alarmas_indicadores-LED.vi" "G3_SAG"() -> (→"G3_SAG":bool)
    n218 = global read "Alarmas_indicadores-LED.vi" "G3_SWELL"() -> (→"G3_SWELL":bool)
    n219 = global read "Alarmas_indicadores-LED.vi" "G3_TRANS"() -> (→"G3_TRANS":bool)
    n220 = global read "Alarmas_indicadores-LED.vi" "G4_TRANS"() -> (→"G4_TRANS":bool)
    n221 = global read "Alarmas_indicadores-LED.vi" "G5_SAG"() -> (→"G5_SAG":bool)
    n222 = global read "Alarmas_indicadores-LED.vi" "G5_SWELL"() -> (→"G5_SWELL":bool)
    n223 = global read "Alarmas_indicadores-LED.vi" "G5_TRANS"() -> (→"G5_TRANS":bool)
    n224 = global read "Alarmas_indicadores-LED.vi" "G6_SAG"() -> (→"G6_SAG":bool)
    n225 = global read "Alarmas_indicadores-LED.vi" "G6_SWELL"() -> (→"G6_SWELL":bool)
    n226 = global read "Alarmas_indicadores-LED.vi" "G6_TRANS"() -> (→"G6_TRANS":bool)
    n227 = global read "Alarmas_indicadores-LED.vi" "G4_SAG"() -> (→"G4_SAG":bool)
    n228 = call "FGV_Stop_Main.vi"("Action"=enum16{"Read", "Write"}."Read") -> ("Error Out"=w334:errorcluster, "Var Out"=w353:bool)  [unwired: 9 in]
    n229 = call "Wait_Main.vi"("Wait time (msec)"=u32 1000 ("milliseconds to wait")) -> ()  [unwired: 5 in]
  }
  n230 = while {
    tunnel: w2 -> [_]
    tunnel: [w357] -> w9
    stop <- w359 stop-if-true
    # "Eventos"
    n231 = call "DB_LeeEventos.vi"() -> ("eventos out"=w356:string)  [unwired: 10 in, 1 out]
    "Eventos" <- w356
    n232 = global write "globalEventos.vi" "Eventos"(w356) -> ()
    n233 = call "FGV_Stop_Main.vi"("Action"=enum16{"Read", "Write"}."Read") -> ("Error Out"=w357:errorcluster, "Var Out"=w359:bool)  [unwired: 9 in]
    n234 = call "Wait_Main.vi"("Wait time (msec)"=u32 1000 ("milliseconds to wait")) -> ()  [unwired: 5 in]
  }
  n235 = Merge Errors(w10, w9, w8, w7, w3) -> (w6:errorcluster)
  n236 = call "Enqueue Error.vi"("error in"=w6) -> ("error out"=w5:errorcluster)  [unwired: 9 in, 1 out]
  n237 = flat-sequence {
    tunnel: w5 -> [_]
    frame #0 {
      n238 = global read "datos usuario.vi" "usuario"() -> (w364:string)
      n239 = call <vilib>:"Space Constant.vi"() -> ("String"=w363:string)
      n240 = Concatenate Strings(w364, w363, "cerró sesión" ("string")) -> (w361:string)
      n241 = call "DB_EscribeTablaEventos.vi"("DESCRIPCION"=w361) -> ()  [unwired: 10 in, 1 out]
    }
    frame #1 {
      n242 = control-ref of="This VI"() -> (w367:refnum<vi>)
      n243 = invoke class="VI" method="FP.Close"(reference=w367) -> (reference out=w365:refnum<vi>, error out=w366:errorcluster)  [unwired: 2 in, 1 out]
      n244 = Close Reference(reference=w365, error in (no error)=w366) -> ()  [unwired: 1 out]
    }
  }
